vi "gpSTS_app.vi"() -> ()   [LabVIEW 2019]
uses:
  <userlib>/Nanonis Prog Interface V45/Nanonis Prog Interface.lvlib
panel:
  out "SpecCurrent":dbl
  out "ScanCurrent":dbl
  out "dpath":path
  out "gpvariance":path
  out "gpmean":path
  out "lastspectra":path
  out "current":path
  out "result":path
  out "command":path
  out "feature":path
  out "Session Path":path
  out "Last Collected Spectrum":picture
  out "Feature":picture
  out "offy":dbl
  out "offx":dbl
  out "Scanning":bool
  in  "Direction: up/down (T=up)":bool=TRUE
  out "Starter Image":picture
  out "driftvar":dbl
  out "ypos":dbl
  out "xpos":dbl
  in  "Write Result":bool
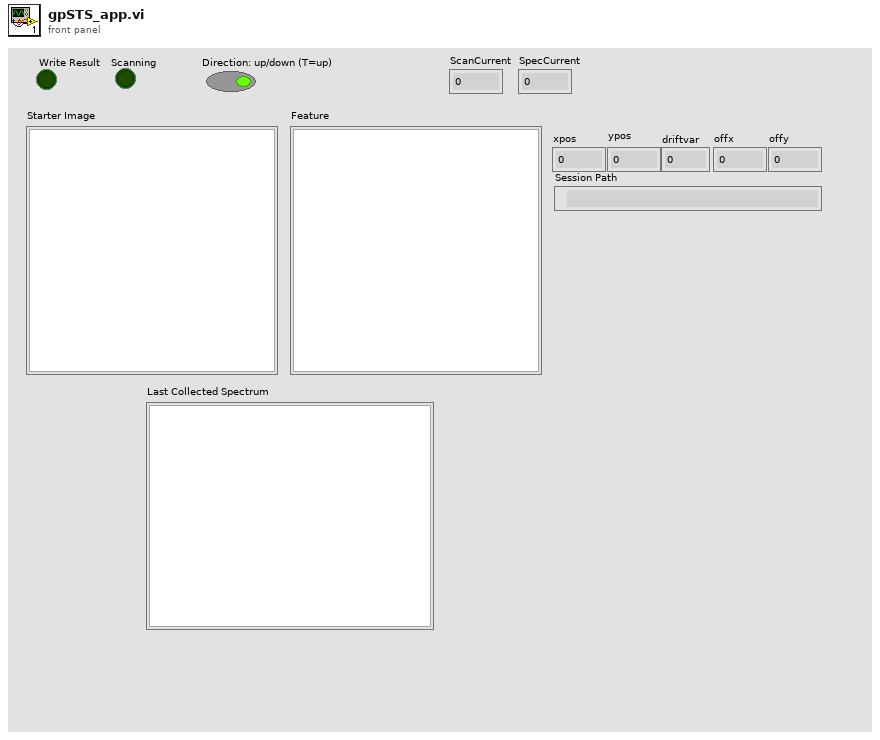
[diagram p1: front panel]
types:
  T1 = cluster{"End settling time (s)":sgl, "Z control time (s)":sgl}
  T2 = cluster{"Z averaging time (s)":sgl, "Z offset (m)":sgl, "Initial settling time (s)":sgl}
  T3 = typedef "imagedata.ctl" = cluster{"image type":i32, "image depth":i32, "image":u8[], "mask":u8[], "colors":u32[], "Rectangle":cluster{"left":i16, "top":i16, "right":i16, "bottom":i16}}
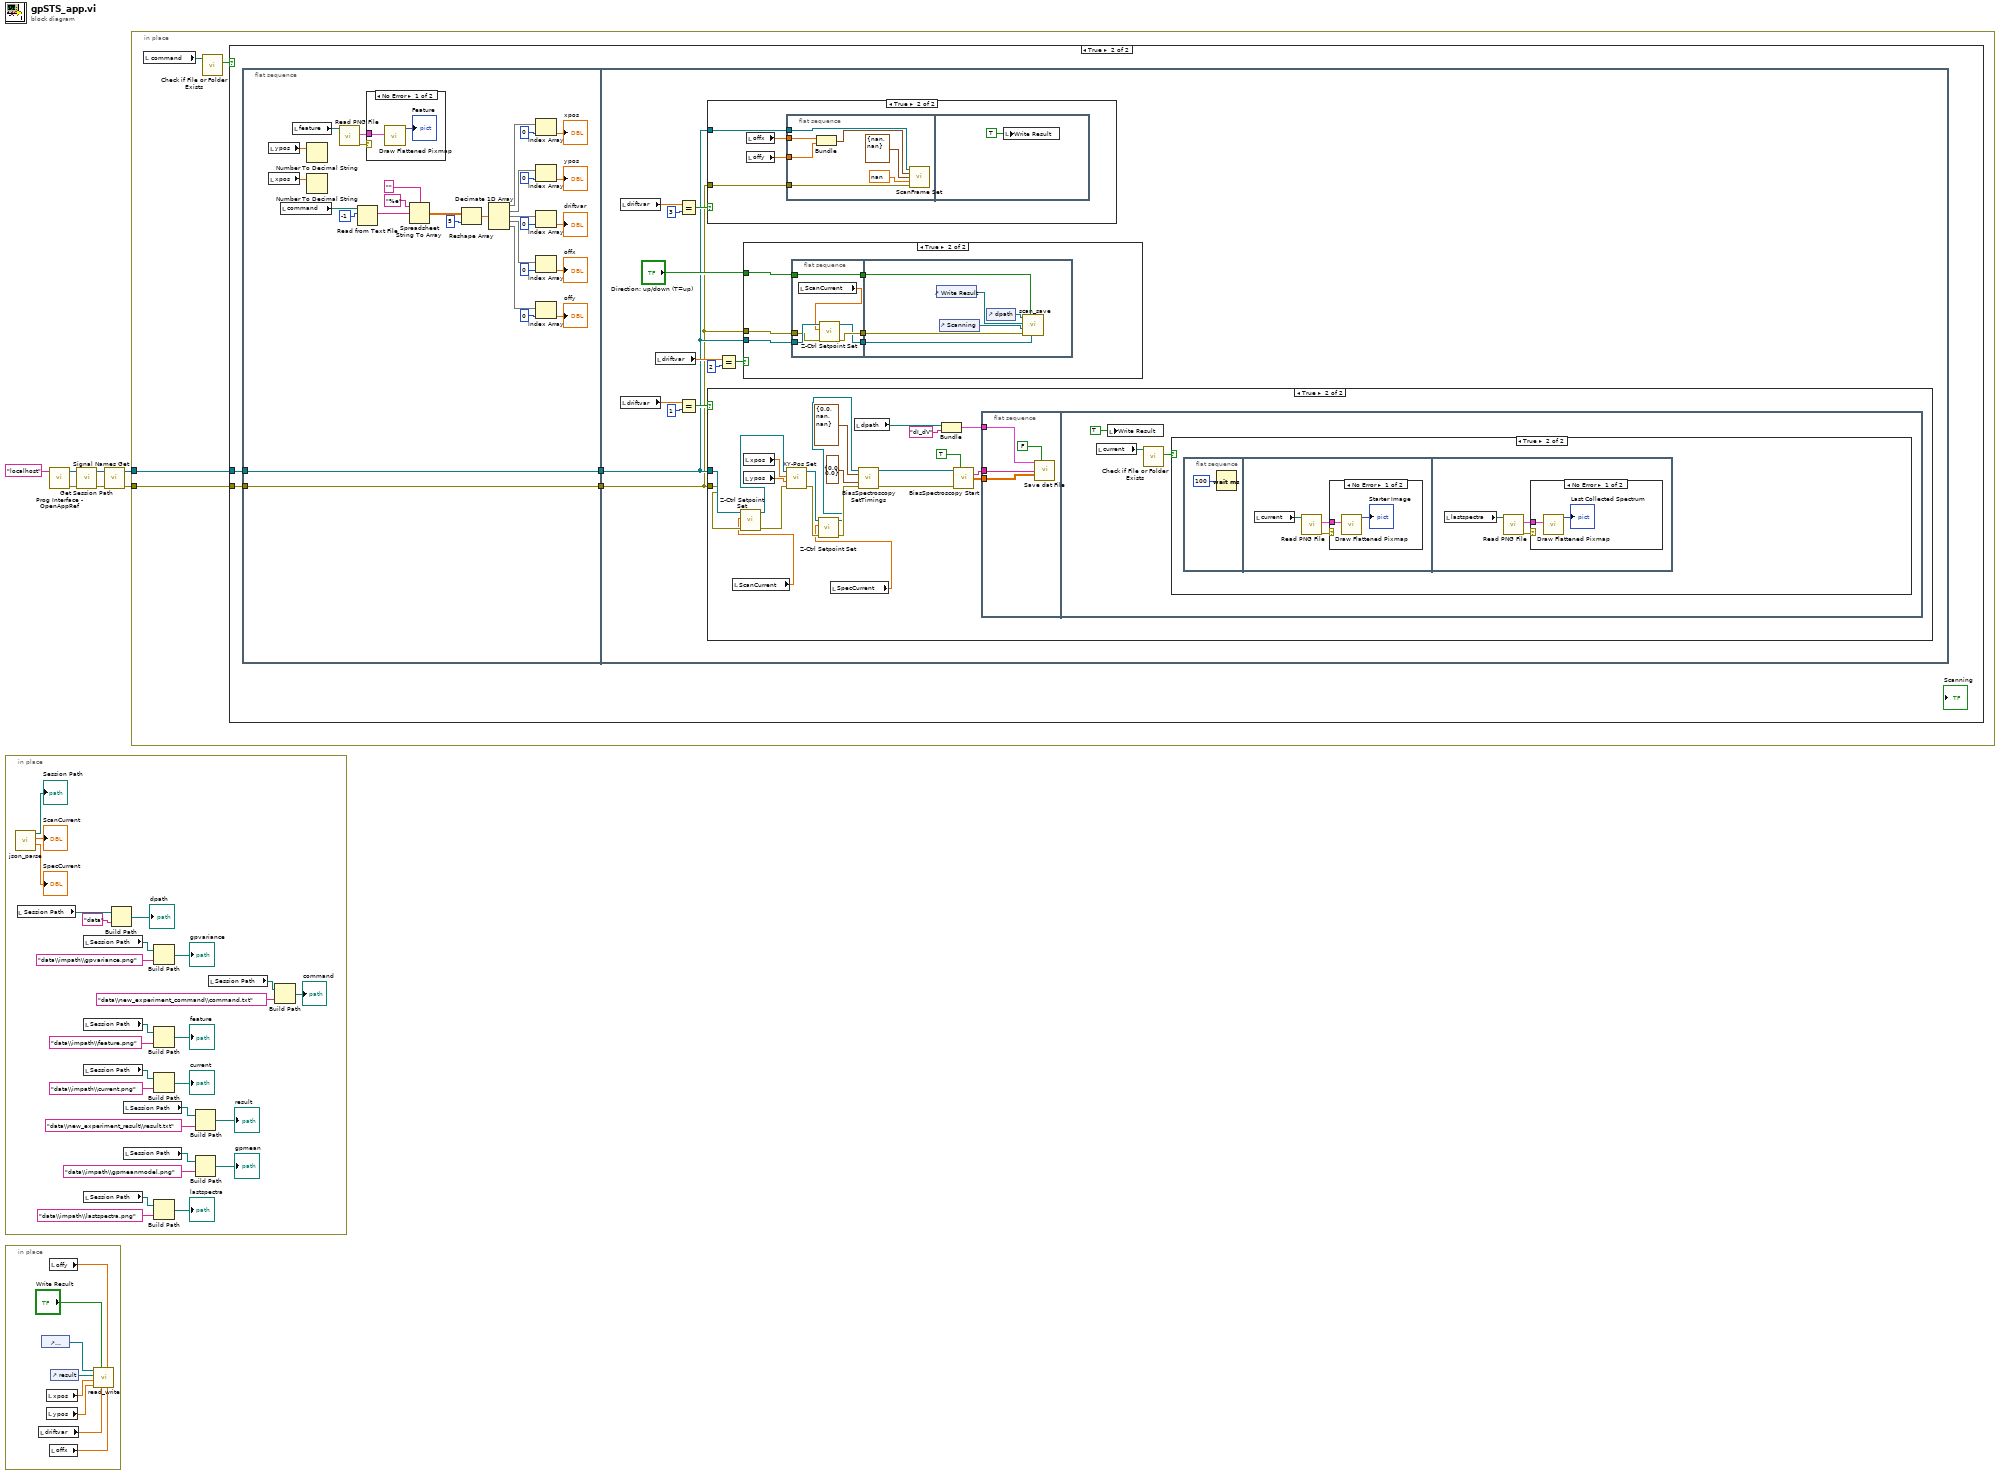
[diagram p0: block diagram]
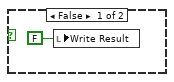
[diagram p2: hidden frame]
diagram:
  n1 = in-place {
    n2 = call "json_parse.vi"() -> ("SpecCurrent"=→"SpecCurrent":dbl, "ScanCurrent"=→"ScanCurrent":dbl, "Path"=→"Session Path":path)  [unwired: 9 in]
    n3 = local read "Session Path"() -> (w17:path)
    n4 = local read "Session Path"() -> (w19:path)
    n5 = local read "Session Path"() -> (w34:path)
    n6 = local read "Session Path"() -> (w25:path)
    n7 = local read "Session Path"() -> (w23:path)
    n8 = Build Path(base path=w17, name or relative path="data") -> (appended path=→"dpath":path)
    n9 = local read "Session Path"() -> (w27:path)
    n10 = local read "Session Path"() -> (w21:path)
    n11 = Build Path(base path=w19, name or relative path="data\\impath\\gpvariance.png") -> (appended path=→"gpvariance":path)
    n12 = Build Path(base path=w34, name or relative path="data\\impath\\feature.png") -> (appended path=→"feature":path)
    n13 = Build Path(base path=w25, name or relative path="data\\impath\\current.png") -> (appended path=→"current":path)
    n14 = Build Path(base path=w23, name or relative path="data\\impath\\lastspectra.png") -> (appended path=→"lastspectra":path)
    n15 = Build Path(base path=w27, name or relative path="data\\new_experiment_result\\result.txt") -> (appended path=→"result":path)
    n16 = Build Path(base path=w21, name or relative path="data\\impath\\gpmeanmodel.png") -> (appended path=→"gpmean":path)
    n17 = local read "Session Path"() -> (w30:path)
    n18 = Build Path(base path=w30, name or relative path="data\\new_experiment_command\\command.txt") -> (appended path=→"command":path)
  }
  n19 = in-place {
    n20 = local read "driftvar"() -> (w39:dbl)
    n21 = control-ref of="command"() -> (w36:refnum<vi>)
    n22 = local read "xpos"() -> (w40:dbl)
    n23 = local read "ypos"() -> (w41:dbl)
    n24 = local read "offy"() -> (w37:dbl)
    n25 = local read "offx"() -> (w38:dbl)
    n26 = control-ref of="result"() -> (w35:refnum<vi>)
    n27 = call "read_write.vi"("offx"=w38, "offy"=w37, "driftvar"=w39, "Write Result"="Write Result", "ypos"=w41, "xpos"=w40, "reference in"=w35, "Path in"=w36) -> ()  [unwired: 4 in]
  }
  n28 = call <userlib>:"Prog Interface - OpenAppRef.vi"("Machine name (local machine IP)"="localhost" ("Machine name (localhost)")) -> ("Error out"=w3:errorcluster, "Application reference"=w6:refnum<vi>)  [unwired: 5 in]
  n29 = call <userlib>:"Get Session Path.vi"("error in (no error)"=w3, "Application ref in"=w6) -> ("error out"=w2:errorcluster, "Application ref out"=w5:refnum<vi>)  [unwired: 7 in, 1 out]
  n30 = call <userlib>:"Signal Names Get.vi"("error in (no error)"=w2, "Application ref in"=w5) -> ("error out"=w1:errorcluster, "Application ref out"=w4:refnum<vi>)  [unwired: 5 in, 1 out]
  n31 = in-place {
    in-place-border: w4 -> [w45]
    in-place-border: w1 -> [w44]
    n32 = local read "command"() -> (w43:path)
    n33 = call <vilib>:"Check if File or Folder Exists.vi"("path"=w43) -> ("file or folder exists?"=w46:bool)  [unwired: 8 in, 2 out]
    n34 = case shown="True" w46 {
      tunnel: w45 -> [_ w50]
      tunnel: w44 -> [_ w51]
      frame False {
        n35 = local write "Write Result"(FALSE ("Boolean")) -> ()
      }
      frame True {
        n36 = flat-sequence {
          tunnel: w50 -> [w57]
          tunnel: w51 -> [w56]
          tunnel: [w57] -> w49
          tunnel: [w56] -> w48
          tunnel: w49 -> [w85]
          tunnel: w48 -> [w84]
          frame #0 {
            n37 = local read "ypos"() -> (w75:dbl)
            n38 = local read "xpos"() -> (w74:dbl)
            n39 = local read "command"() -> (w53:path)
            n40 = local read "feature"() -> (w52:path)
            n41 = Number To Decimal String(number=w75) -> ()  [unwired: 1 in, 1 out]
            n42 = Number To Decimal String(number=w74) -> ()  [unwired: 1 in, 1 out]
            n43 = call <vilib>:"Read PNG File.vi"("path to PNG file"=w52) -> ("error out"=w55:errorcluster, "image data"=w54:T3)  [unwired: 8 in, 1 out]
            n44 = Read from Text File(file (use dialog)=w53, count=-1) -> (text=w68:string)  [unwired: 2 in, 3 out]
            n45 = case shown="No Error" w55 {
              tunnel: w54 -> [w82 _]
              frame No Error {
                n46 = call <vilib>:"Draw Flattened Pixmap.vi"("image data"=w82) -> ("new picture"=→"Feature":picture)  [unwired: 8 in]
              }
              frame Error {
              }
            }
            n47 = Spreadsheet String To Array(delimiter (Tab)="", format string="%e", spreadsheet string=w68) -> (array=w67:dbl[][])  [unwired: 1 in]
            n48 = Reshape Array(w67, 5 ("dimension size")) -> (w69:dbl[])
            n49 = Decimate 1D Array(w69) -> (w70:dbl[], w71:dbl[], w76:dbl[], w78:dbl[], w79:dbl[])
            n50 = Index Array(array=w70, index=0) -> (element=→"xpos":dbl)
            n51 = Index Array(array=w71, index=0) -> (element=→"ypos":dbl)
            n52 = Index Array(array=w76, index=0) -> (element=→"driftvar":dbl)
            n53 = Index Array(array=w78, index=0) -> (element=→"offx":dbl)
            n54 = Index Array(array=w79, index=0) -> (element=→"offy":dbl)
          }
          frame #1 {
            n55 = local read "driftvar"() -> (w88:dbl)
            n56 = local read "driftvar"() -> (w95:dbl)
            n57 = local read "driftvar"() -> (w91:dbl)
            n58 = Equal?(x=w88, y=3 ("index")) -> (x = y?=w86:bool)
            n59 = Equal?(x=w95, y=1 ("index")) -> (x = y?=w93:bool)
            n60 = case shown="True" w86 {
              tunnel: w85 -> [_ w99]
              tunnel: w84 -> [_ w98]
              frame False {
              }
              frame True {
                n61 = local read "offx"() -> (w97:dbl)
                n62 = local read "offy"() -> (w96:dbl)
                n63 = flat-sequence {
                  tunnel: w99 -> [w106]
                  tunnel: w98 -> [w105]
                  tunnel: w97 -> [w101]
                  tunnel: w96 -> [w100]
                  frame #0 {
                    n64 = Bundle("offx"=w101, "offy"=w100) -> (w104:cluster{"offx":dbl, "offy":dbl})  [unwired: 1 in]
                    n65 = call <userlib>:"ScanFrame Set.vi"("Application ref in"=w106, "Center coordinates (m)"=w104, "Size (m)"=cluster{"Width":sgl, "Height":sgl} {"Width"=nan, "Height"=nan}, "Angle (deg)"=sgl nan, "error in (no error)"=w105) -> ()  [unwired: 9 in, 2 out]
                  }
                  frame #1 {
                    n66 = local write "Write Result"(TRUE ("Write Result")) -> ()
                  }
                }
              }
            }
            n67 = case shown="True" w93 {
              tunnel: w85 -> [_ w137]
              tunnel: w84 -> [_ w135]
              frame False {
              }
              frame True {
                n68 = local read "ScanCurrent"() -> (w129:dbl)
                n69 = call <userlib>:"Z-Ctrl Setpoint Set.vi"("error in (no error)"=w135, "Z Controller setpoint"=w129, "Application ref in"=w137) -> ("error out"=w134:errorcluster, "Application ref out"=w136:refnum<vi>)  [unwired: 7 in]
                n70 = local read "xpos"() -> (w140:dbl)
                n71 = local read "ypos"() -> (w139:dbl)
                n72 = call <userlib>:"XY-Pos Set.vi"("error in (no error)"=w134, "Y (m)"=w139, "X (m)"=w140, "Application ref in"=w136) -> ("error out"=w133:errorcluster, "Application ref out"=w132:refnum<vi>)  [unwired: 4 in]
                n73 = local read "SpecCurrent"() -> (w128:dbl)
                n74 = call <userlib>:"Z-Ctrl Setpoint Set.vi"("error in (no error)"=w133, "Z Controller setpoint"=w128, "Application ref in"=w132) -> ("error out"=w131:errorcluster, "Application ref out"=w130:refnum<vi>)  [unwired: 7 in]
                n75 = local read "dpath"() -> (w138:path)
                n76 = call <userlib>:"BiasSpectroscopy SetTimings.vi"("Application ref in"=w130, "Initialization (NaN)"=T2 {"Z averaging time (s)"=0.0, "Z offset (m)"=nan, "Initial settling time (s)"=nan}, "End of Sweep (NaN)"=T1 {"End settling time (s)"=0.0, "Z control time (s)"=0.0}, "Error in (no error)"=w131) -> ("Application ref out"=w127:refnum<vi>, "Error out"=w126:errorcluster)  [unwired: 10 in]
                n77 = Bundle("dpath"=w138, "Basename"="dI_dV") -> (w145:cluster{"dpath":path, "Basename":string})  [unwired: 1 in]
                n78 = call <userlib>:"BiasSpectroscopy Start.vi"("Application ref in"=w127, "Get data (F)"=TRUE, "Error in (no error)"=w126) -> ("Channels"=w141:string[], "Data"=w142:sgl[][])  [unwired: 8 in, 3 out]
                n79 = flat-sequence {
                  tunnel: w142 -> [w150]
                  tunnel: w145 -> [w151]
                  tunnel: w141 -> [w148]
                  frame #0 {
                    n80 = call <userlib>:"Save dat File.vi"("Filename control"=w151, "Show save dialog (T)"=FALSE, "Channels names"=w148, "Data"=w150) -> ()  [unwired: 8 in, 4 out]
                  }
                  frame #1 {
                    n81 = local read "current"() -> (w152:path)
                    n82 = local write "Write Result"(TRUE ("Boolean")) -> ()
                    n83 = call <vilib>:"Check if File or Folder Exists.vi"("path"=w152) -> ("file or folder exists?"=w153:bool)  [unwired: 8 in, 2 out]
                    n84 = case shown="True" w153 {
                      frame False {
                      }
                      frame True {
                        n85 = flat-sequence {
                          frame #0 {
                            n86 = Wait (ms)(milliseconds to wait=u32 100 ("millisecond timer value")) -> ()  [unwired: 1 out]
                          }
                          frame #1 {
                            n87 = local read "current"() -> (w156:path)
                            n88 = call <vilib>:"Read PNG File.vi"("path to PNG file"=w156) -> ("error out"=w158:errorcluster, "image data"=w157:T3)  [unwired: 8 in, 1 out]
                            n89 = case shown="No Error" w158 {
                              tunnel: w157 -> [w159 _]
                              frame No Error {
                                n90 = call <vilib>:"Draw Flattened Pixmap.vi"("image data"=w159) -> ("new picture"=→"Starter Image":picture)  [unwired: 8 in]
                              }
                              frame Error {
                              }
                            }
                          }
                          frame #2 {
                            n91 = local read "lastspectra"() -> (w161:path)
                            n92 = call <vilib>:"Read PNG File.vi"("path to PNG file"=w161) -> ("error out"=w163:errorcluster, "image data"=w162:T3)  [unwired: 8 in, 1 out]
                            n93 = case shown="No Error" w163 {
                              tunnel: w162 -> [w164 _]
                              frame No Error {
                                n94 = call <vilib>:"Draw Flattened Pixmap.vi"("image data"=w164) -> ("new picture"=→"Last Collected Spectrum":picture)  [unwired: 8 in]
                              }
                              frame Error {
                              }
                            }
                          }
                        }
                      }
                    }
                  }
                }
              }
            }
            n95 = Equal?(x=w91, y=2 ("index")) -> (x = y?=w89:bool)
            n96 = case shown="True" w89 {
              tunnel: w85 -> [_ w112]
              tunnel: w84 -> [_ w113]
              tunnel: "Direction: up/down (T=up)" -> [_ w111]
              frame False {
              }
              frame True {
                n97 = flat-sequence {
                  tunnel: w111 -> [w119]
                  tunnel: w112 -> [w118]
                  tunnel: w113 -> [w117]
                  tunnel: [w116] -> w110
                  tunnel: [w115] -> w109
                  tunnel: [w119] -> w108
                  tunnel: w110 -> [w125]
                  tunnel: w109 -> [w124]
                  tunnel: w108 -> [w123]
                  frame #0 {
                    n98 = local read "ScanCurrent"() -> (w114:dbl)
                    n99 = call <userlib>:"Z-Ctrl Setpoint Set.vi"("error in (no error)"=w117, "Z Controller setpoint"=w114, "Application ref in"=w118) -> ("error out"=w116:errorcluster, "Application ref out"=w115:refnum<vi>)  [unwired: 7 in]
                  }
                  frame #1 {
                    n100 = control-ref of="Write Result"() -> (w121:refnum<vi>)
                    n101 = control-ref of="Scanning"() -> (w120:refnum<vi>)
                    n102 = control-ref of="dpath"() -> (w122:refnum<vi>)
                    n103 = call "scan_save.vi"("Application ref in"=w124, "Direction: up/down (T=up)"=w123, "error in (no error)"=w125, "reference 3"=w120, "reference in"=w121, "Path in"=w122) -> ()  [unwired: 6 in]
                  }
                }
              }
            }
          }
        }
      }
    }
  }
